vi "Update Table Add Tasks.vi"(6 "Digital Acquisition Parameters":T1 {"Execution Task Frequency" scale=1.0..100.0}, 7 "Analog Acquisition Parameters":T2={"sampling frequency Analog"=1000, "number of samples Analog"=1000, "Channels Analog"=[]} {"number of samples Analog" scale=0.0..2000.0; "sampling frequency Analog" scale=0.0..2000.0}, 8 "error in (no error)":errorcluster, 9 "Total Acquisition Time":i32, 10 "DAQ Device Name":tag, 11 "Analog - Digital":bool) -> (0 "error out":errorcluster)   [LabVIEW 2020, in "Settings.lvlib"]
uses:
  Settings.lvlib
  Shared/AnalogAcquisitionParameters__typedef.ctl
  Shared/DigitalAcquisitionParameters__typedef.ctl
  <vilib>/drjdpowell/SQLite Library/SQL Connection/Open (path).vi
  <vilib>/drjdpowell/SQLite Library/SQL Connection/Open (string).vi
  <vilib>/AdvancedString/Path To Command Line String.vi
  <vilib>/drjdpowell/SQLite Library/SQL Connection/Execute SQL (No results).vi
  <vilib>/drjdpowell/SQLite Library/SQL Connection/Connection.lvclass
  <vilib>/drjdpowell/SQLite Library/SQLite.lvlib
  Shared/Configuration for Acquisitions.lvlib
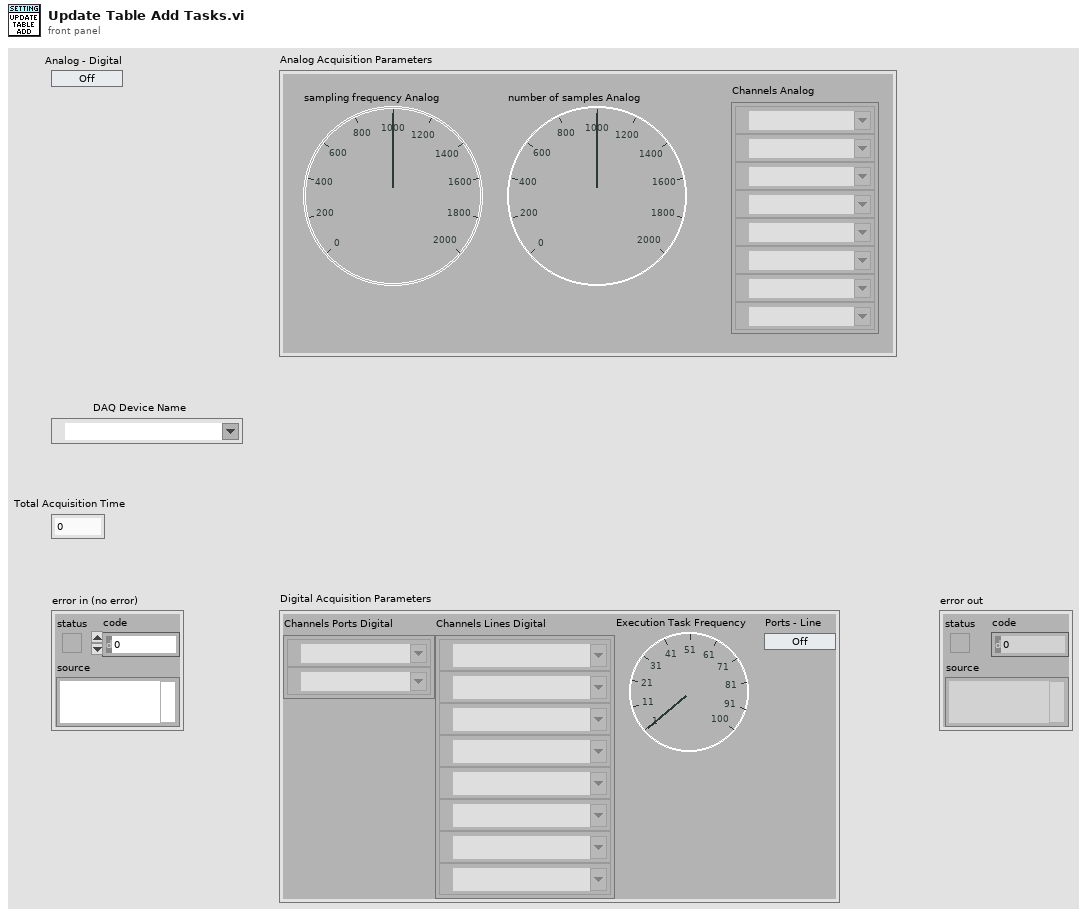
[diagram p1: front panel]
types:
  T1 = typedef "Configuration for Acquisitions.lvlib/DigitalAcquisitionParameters__typedef.ctl" = cluster{"Channels Ports Digital":tag[], "Channels Lines Digital":tag[], "Execution Task Frequency\n":u32, "Ports - Line":bool}
  T2 = typedef "Configuration for Acquisitions.lvlib/AnalogAcquisitionParameters__typedef.ctl" = cluster{"sampling frequency Analog":u32, "number of samples Analog":u32, "Channels Analog":tag[]}
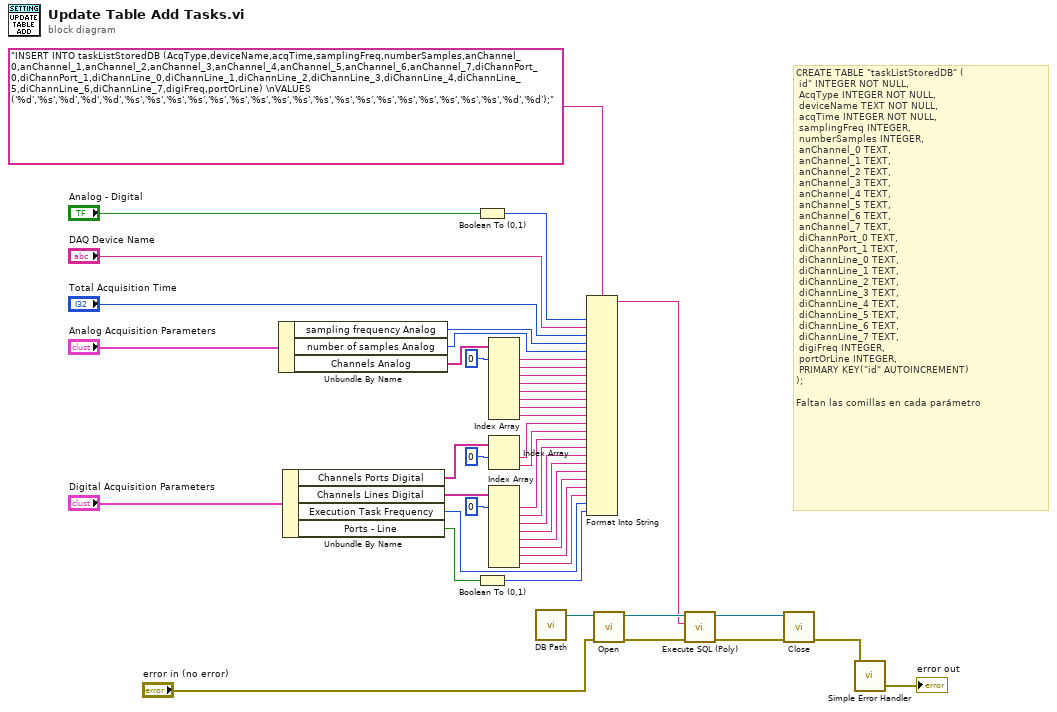
[diagram p0: block diagram]
diagram:
  # "CREATE TABLE \"taskListStoredDB\" (\n\tid\"\tINTEGER NOT NULL,\n\tAcqType\tINTEGER NOT NULL,\n\tdeviceName\tTEXT NOT NULL,\n\tacqTime\tINTEGER NOT NULL,\n\tsamplingFreq\tINTEGER,\n\tnumberSamples\tINTEGER,\n\tanChannel_0\tTEXT,\n\tanChannel_1\tTEXT,\n\tanChannel_2\tTEXT,\n\tanChannel_3\tTEXT,\n\tanChannel_4 TEXT,\n\tanChannel_5\tTEXT,\n\tanChannel_6\tTEXT,\n\tanChannel_7\tTEXT,\n\tdiChannPort_0\tTEXT,\n\tdiChannPort_1\tTEXT,\n\tdiChannLine_0\tTEXT,\n\tdiChannLine_1\tTEXT,\n\tdiChannLine_2\tTEXT,\n\tdiChannLine_3\tTEXT,\n\tdiChannLine_4\tTEXT,\n\tdiChannLine_5\tTEXT,\n\tdiChannLine_6\tTEXT,\n\tdiChannLine_7\tTEXT,\n\tdigiFreq\tINTEGER,\n\tportOrLine INTEGER,\n\tPRIMARY KEY(\"id\" AUTOINCREMENT)\n);\n\nFaltan las comillas en cada parámetro"
  n1 = Unbundle By Name("Analog Acquisition Parameters") -> ("sampling frequency Analog"=w39:u32, "number of samples Analog"=w38:u32, "Channels Analog"=w36:tag[])
  n2 = Unbundle By Name("Digital Acquisition Parameters") -> ("Channels Ports Digital"=w25:tag[], "Channels Lines Digital"=w21:tag[], "Execution Task Frequency"=w12:u32, "Ports - Line"=w11:bool)
  n3 = Boolean To (0,1)(Boolean="Analog - Digital") -> (0, 1=w43:i16)
  n4 = Boolean To (0,1)(Boolean=w11) -> (0, 1=w10:i16)
  n5 = Index Array(array=w36, index #1=0 ("index")) -> (element #1=w35:tag, element #2=w34:tag, element #3=w33:tag, element #4=w32:tag, element #5=w31:tag, element #6=w30:tag, element #7=w29:tag, element #8=w28:tag)  [unwired: 7 in]
  n6 = Index Array(array=w25, index #1=0 ("index")) -> (element #1=w24:tag, element #2=w23:tag)  [unwired: 1 in]
  n7 = Index Array(array=w21, index #1=0 ("index")) -> (element #1=w20:tag, element #2=w19:tag, element #3=w18:tag, element #4=w17:tag, element #5=w16:tag, element #6=w15:tag, element #7=w14:tag, element #8=w13:tag)  [unwired: 7 in]
  n8 = call "DB Path.vi"() -> ("DB Path"=w4:path)  [unwired: 11 in]
  n9 = Format Into String(format string="INSERT INTO taskListStoredDB (AcqType,deviceName,acqTime,samplingFreq,numberSamples,anChannel_0,anChannel_1,anChannel_2,anChannel_3,anChannel_4,anChannel_5,anChannel_6,anChannel_7,diChannPort_0,diChannPort_1,diChannLine_0,diChannLine_1,diChannLine_2,diChannLine_3,diChannLine_4,diChannLine_5,diChannLine_6,diChannLine_7,digiFreq,portOrLine) \nVALUES ('%d','%s','%d','%d','%d','%s','%s','%s','%s','%s','%s','%s','%s','%s','%s','%s','%s','%s','%s','%s','%s','%s','%s','%d','%d');", w43, "DAQ Device Name", "Total Acquisition Time", w39, w38, w35, w34, w33, w32, w31, w30, w29, w28, w24, w23, w20, w19, w18, w17, w16, w15, w14, w13, w12, w10) -> (resulting string=w3:string)  [unwired: 2 in, 1 out]
  n10 = call-poly <vilib>:"Open.vi"("error in (no error)"="error in (no error)", "db file"=w4) -> ("error out"=w9:errorcluster, "SQLite Connection"=w6:refnum<class "Connection.lvclass">)  [unwired: 8 in]
  n11 = call-poly <vilib>:"Execute SQL (Poly).vi"("error in (no error)"=w9, "SQL"=w3, "SQLite Connection in"=w6) -> ("error out"=w7:errorcluster, "SQLite Connection"=w8:refnum<class "Connection.lvclass">)  [unwired: 7 in]
  n12 = call-dynamic "Close.vi"("error in (no error)"=w7, "SQLite Connection in"=w8) -> ("error out"=w2:errorcluster)  [unwired: 9 in]
  n13 = call <vilib>:"Simple Error Handler.vi"("error in (no error)"=w2) -> ("error out"=→"error out":errorcluster)  [unwired: 4 in, 4 out]
